vi "FT Read GPIO.vi"(8 "error in (no error)":errorcluster, 11 "handle":u32) -> (0 "error out":errorcluster, 2 "value out":string, 3 "handle out":u32)   [LabVIEW 2018, in "libMPSSE-SPI.lvlib"]
doc: "FTDI_API FT_STATUS FT_ReadGPIO(FT_HANDLE handle,uint8 *value);"
uses:
  libMPSSE-SPI.lvlib
  dll/libMPSSE.dll
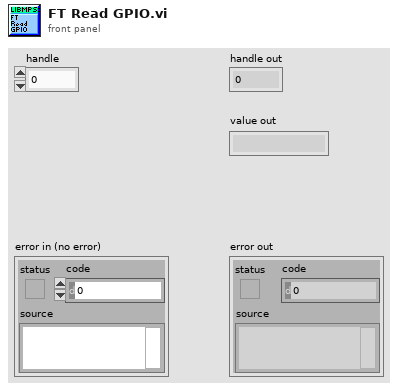
[diagram p1: front panel]
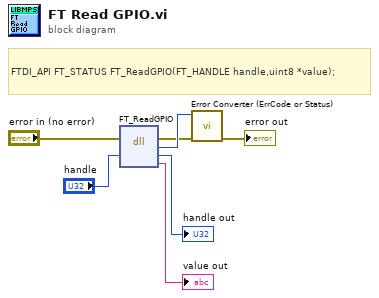
[diagram p0: block diagram]
diagram:
  # "FTDI_API FT_STATUS FT_ReadGPIO(FT_HANDLE handle,uint8 *value);"
  n1 = dll-call lib="D:/LABVIEW/Examples - 32bit/FTDI/libMPSSE-SPI-LabVIEW-master/dll/libMPSSE.*" fn="FT_ReadGPIO"(error in="error in (no error)", "handle"="handle") -> (error out=w2:errorcluster, w7:u32, "handle"=→"handle out":u32, "value"=→"value out":string)  [unwired: 3 in, 1 out]
  n2 = call "Error Converter (ErrCode or Status).vi"("error in (no error)"=w2, "error code"=w7) -> ("error out"=→"error out":errorcluster)  [unwired: 9 in]
